vi "FGV Scan List Data.vi"(7 "Wavelength Scan List Actions":T2=enum."Import from file", 8 "Error In":errorcluster, 11 "Wavelength Scan List IN":T1[](array[typedef]) {"Setpoint Wavelength" format="%.4f"}) -> (0 "Error Out":errorcluster, 3 "Wavelength Scan List OUT":T1[](array[typedef]) {"Setpoint Wavelength" format="%.4f"})   [LabVIEW 2013]
uses:
  Type Definitions/Type Setpoint Info.ctl
  Type Definitions/Type Wavelength Scan List Actions.ctl
  <vilib>/Utility/file.llb/Read From Spreadsheet File (DBL).vi
  <vilib>/Utility/file.llb/Write To Spreadsheet File (DBL).vi
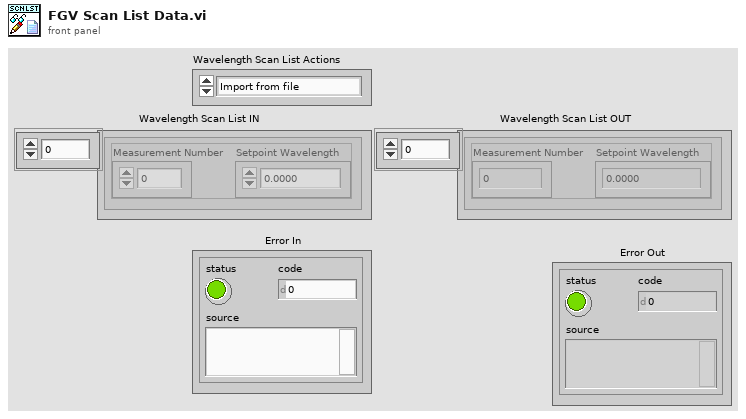
[diagram p1: front panel]
types:
  T1 = typedef "Type Setpoint Info.ctl" = cluster{"Measurement Number":i32, "Setpoint Wavelength":dbl}
  T2 = typedef "Type Wavelength Scan List Actions.ctl" = enum16{"Init", "Import from file", "Export to file", "Read", "Write", "Update"}
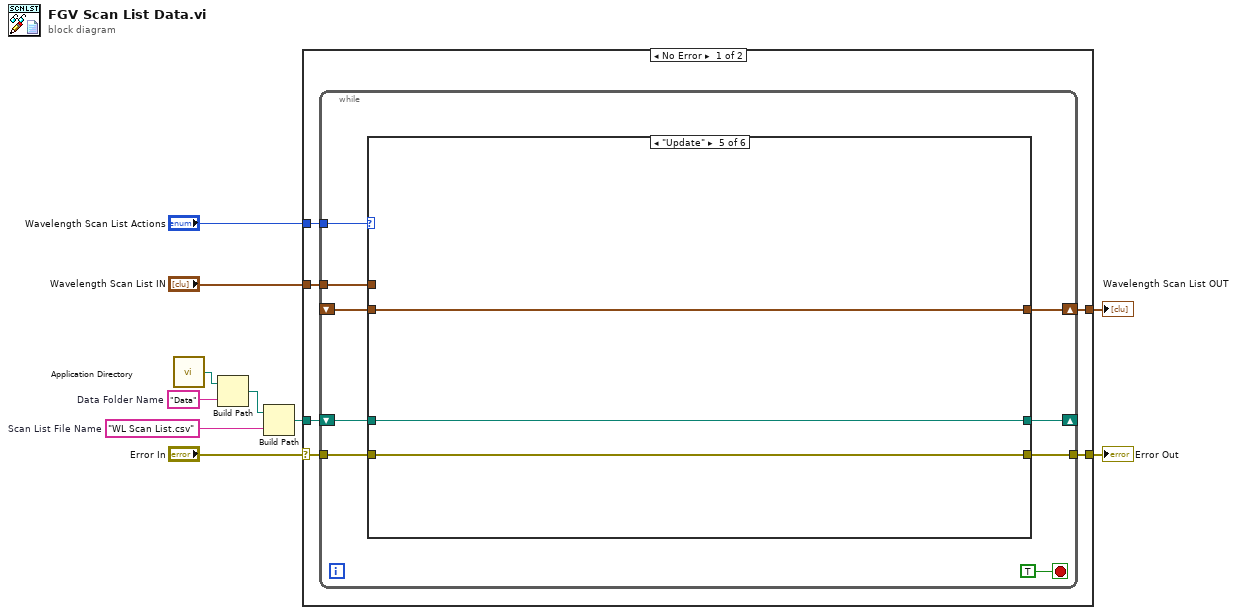
[diagram p0: block diagram]
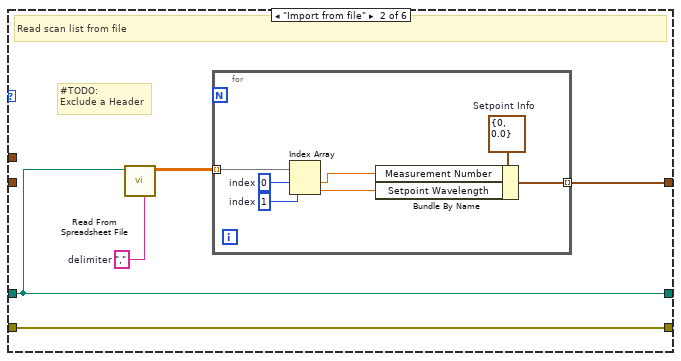
[diagram p3: hidden frame]
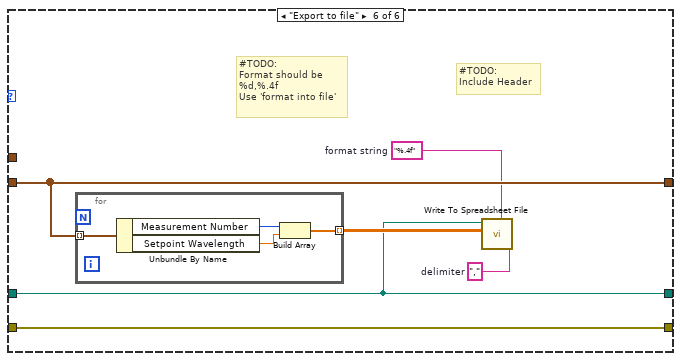
[diagram p6: hidden frame]
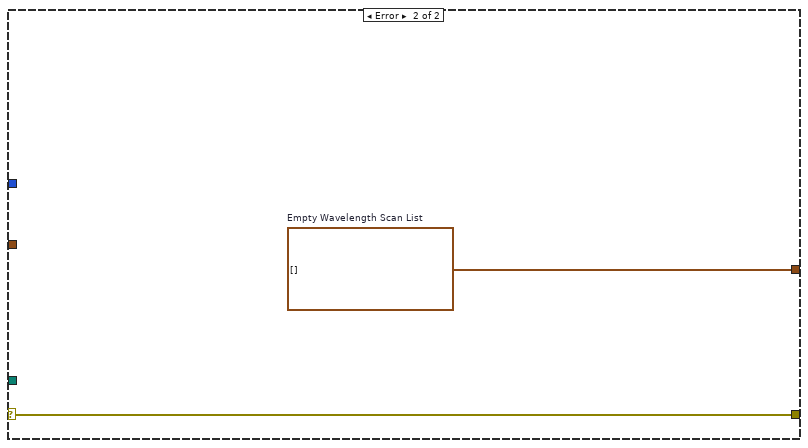
[diagram p7: hidden frame]
diagram:
  w6 = "WL Scan List.csv"  # Scan List File Name
  w7 = "Data"  # Data Folder Name
  n1 = call <vilib>:"Application Directory.vi"() -> ("Application Directory"=w8:path)
  n2 = Build Path(base path=w8, name or relative path=w7) -> (appended path=w5:path)
  n3 = Build Path(base path=w5, name or relative path=w6) -> (appended path=w4:path)
  n4 = case shown="No Error" "Error In" {
    selector: "Error In" -> [w12 w61]
    tunnel: [w16 w60] -> w10
    tunnel: "Wavelength Scan List Actions" -> [w15 _]
    tunnel: w4 -> [w14 _]
    tunnel: "Wavelength Scan List IN" -> [w13 _]
    tunnel: [w11 w61] -> w1
    frame No Error {
      n5 = while {
        tunnel: w15 -> [w24]
        shift-right: [w22] -> w16
        shift-left: _ -> [w21]
        shift-right: [w20] -> _
        shift-left: w14 -> [w23]
        tunnel: w13 -> [w19]
        tunnel: [w18] -> w11
        tunnel: w12 -> [w17]
        stop <- TRUE stop-if-true
        n6 = case shown="\"Update\"" w24 {
          tunnel: w23 -> [w27 w33 w43 w46 w48 w51]
          tunnel: [w28 w31 w41 w44 w49 w55] -> w22
          tunnel: w21 -> [w28 _ w41 _ w49 w55]
          tunnel: [w27 w33 w43 w46 w48 w51] -> w20
          tunnel: w19 -> [_ _ _ w44 _ _]
          tunnel: [w26 w29 w42 w45 w47 w54] -> w18
          tunnel: w17 -> [w26 w29 w42 w45 w47 w54]
          frame "Init", Default {
            # "Save file reference to FGV"
          }
          frame "Import from file" {
            w30 = ","  # delimiter
            # "#TODO:\nExclude a Header"
            # "Read scan list from file"
            n7 = call-poly <vilib>:"Read From Spreadsheet File.vi"("delimiter (\\t)"=w30, "file path (dialog if empty)"=w33) -> ("all rows"=w32:dbl[][])  [unwired: 5 in, 4 out]
            n8 = for {
              tunnel: w32 -> [w40] mode=indexing
              tunnel: [w36] -> w31 mode=indexing
              w34 = 1  # index
              w35 = 0  # index
              w39 = T1 {"Measurement Number"=0, "Setpoint Wavelength"=0.0}  # Setpoint Info
              n9 = Index Array(array=w40, index #1=w35, index #2=w34) -> (element #1=w38:dbl, element #2=w37:dbl)
              n10 = Bundle By Name(cluster=w39, "Measurement Number"=w38, "Setpoint Wavelength"=w37) -> (w36:T1)
            }
          }
          frame "Read" {
          }
          frame "Write" {
          }
          frame "Update" {
          }
          frame "Export to file" {
            w50 = ","  # delimiter
            w52 = "%.4f"  # format string
            # "#TODO:\nInclude Header"
            # "#TODO:\nFormat should be\n%d,%.4f\nUse 'format into file'"
            n11 = for {
              tunnel: w55 -> [w59] mode=indexing
              tunnel: [w56] -> w53 mode=indexing
              n12 = Unbundle By Name(w59) -> ("Measurement Number"=w58:i32, "Setpoint Wavelength"=w57:dbl)
              n13 = Build Array(w58, w57) -> (w56:dbl[])
            }
            n14 = call-poly <vilib>:"Write To Spreadsheet File.vi"("delimiter (\\t)"=w50, "format (%.3f)"=w52, "2D data"=w53, "file path (dialog if empty)"=w51) -> ()  [unwired: 4 in, 1 out]
          }
        }
      }
    }
    frame Error {
      w60 = T1[] []  # Empty Wavelength Scan List
    }
  }
  "Wavelength Scan List OUT" <- w10
  "Error Out" <- w1
